vi "UI.ManagePropertiesView.vi"(8 "error in (no error)":errorcluster, 10 "NewVal":T4, 11 "State Variables":T1={"Aliases.All"=[], "Aliases.Outputs"=[], "UI.Sequence#ofColumns"=0, "SysDef.Path"=path "", "UI.SequenceRef"=refnum, "UI.StepInformationRef"=refnum, "UI.AbortRef"=refnum, "UI.GraphRef"=refnum, "UI.ViewRef"=refnum, "UI.IterationsRef"=refnum, "UI.IterationInformationRef"=refnum, "INI.Settings"={"Build Location"=path "C:/Simple Sequence Editor/SequenceRepo", "LoggingLocation"=path ""}, "NIVS.Workspace Event"=refnum, "UI.SkipChannel"=refnum, "NIVS.Launched?"=FALSE, "UI.DurationChannel"=refnum}) -> (0 "error out":errorcluster)   [LabVIEW 2015, in "Simple Sequence Tools - Editor.lvlib"]
uses:
  Simple Sequence Tools - Editor.lvlib
  Types/UI.PropertiesTypes.ctl
  Types/Main.StateVariables.ctl
  Shared/Types/Channel.Properties.ctl
  Shared/Types/INI.Settings
  Shared/Simple Sequence Tools - Shared.lvlib
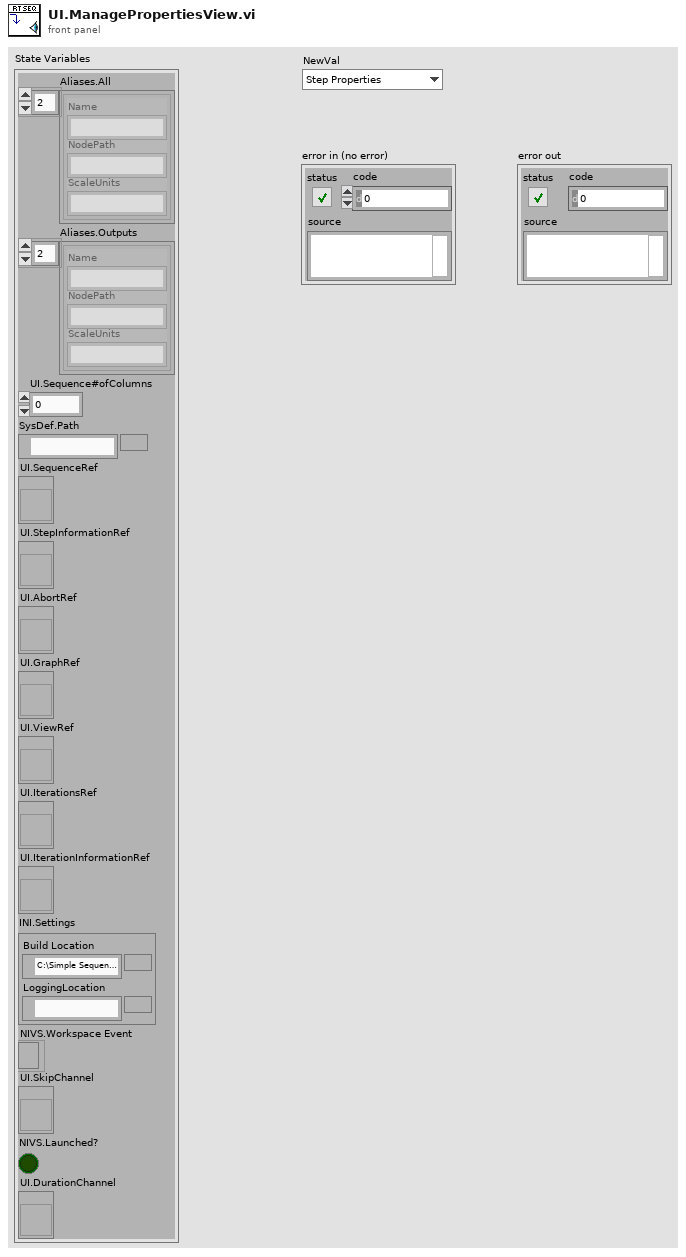
[diagram p1: front panel]
types:
  T1 = typedef "Simple Sequence Tools - Editor.lvlib/Main.StateVariables.ctl" = cluster{"Aliases.All":T2[], "Aliases.Outputs":T2[], "UI.Sequence#ofColumns":i32, "SysDef.Path":path, "UI.SequenceRef":refnum<vi>, "UI.StepInformationRef":refnum<vi>, "UI.AbortRef":refnum<vi>, "UI.GraphRef":refnum<vi>, "UI.ViewRef":refnum<vi>, "UI.IterationsRef":refnum<vi>, "UI.IterationInformationRef":refnum<vi>, "INI.Settings":T3, "NIVS.Workspace Event":refnum<event-registration>, "UI.SkipChannel":refnum<vi>, "NIVS.Launched?":bool, "UI.DurationChannel":refnum<vi>}
  T2 = typedef "Simple Sequence Tools - Shared.lvlib/Channel.Properties.ctl" = cluster{"Name":string, "NodePath":string, "ScaleUnits":string}
  T3 = typedef "Simple Sequence Tools - Shared.lvlib/INI.Settings" = cluster{"Build Location":path, "LoggingLocation":path}
  T4 = typedef "Simple Sequence Tools - Editor.lvlib/UI.PropertiesTypes.ctl" = enum8{"Step Properties", "Sequence Properties"}
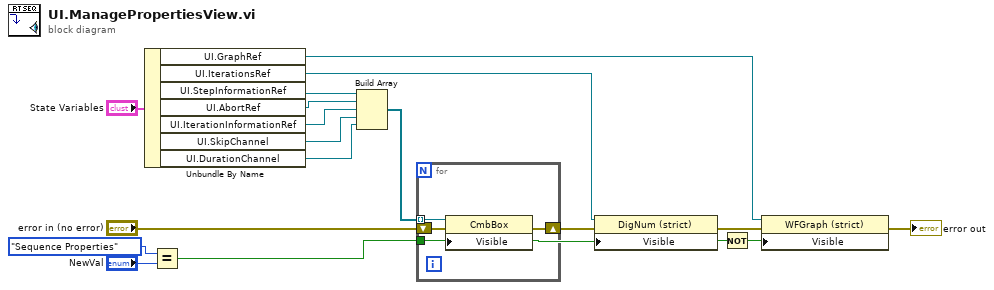
[diagram p0: block diagram]
diagram:
  n1 = Unbundle By Name("State Variables") -> ("UI.GraphRef"=w11:refnum<vi>, "UI.IterationsRef"=w13:refnum<vi>, "UI.StepInformationRef"=w4:refnum<vi>, "UI.AbortRef"=w5:refnum<vi>, "UI.IterationInformationRef"=w17:refnum<vi>, "UI.SkipChannel"=w2:refnum<vi>, "UI.DurationChannel"=w1:refnum<vi>)
  n2 = Equal?(x=UI.PropertiesTypes."Sequence Properties" ("View"), y="NewVal") -> (x = y?=w16:bool)
  n3 = Build Array(w4, w5, w17, w2, w1) -> (w6:refnum<vi>[])
  n4 = for {
    tunnel: w6 -> [w21] mode=indexing
    shift-right: [w19] -> w14
    shift-left: "error in (no error)" -> [w20]
    tunnel: w16 -> [w18]
    n5 = property class="CmbBox"(reference=w21, error in=w20, "Visible"=w18) -> (error out=w19:errorcluster)  [unwired: 1 out]
  }
  n6 = property class="DigNum (strict)"(reference=w13, error in=w14, "Visible"=w16) -> (error out=w15:errorcluster)  [unwired: 1 out]
  n7 = Not(x=w16) -> (.not. x?=w12:bool)
  n8 = property class="WFGraph (strict)"(reference=w11, error in=w15, "Visible"=w12) -> (error out=→"error out":errorcluster)  [unwired: 1 out]
